vi "EXA_Get_Marker_Value.vi"(8 "error in":errorcluster, 10 "Marker\nNumber":i32, 11 "VISA resource name":refnum<visa-resource-name>) -> (0 "error out":errorcluster, 1 "Amplitude (dBm)":dbl, 2 "Frequency (Hz)":dbl, 3 "VISA resource name":refnum<visa-resource-name>)   [LabVIEW 2016]
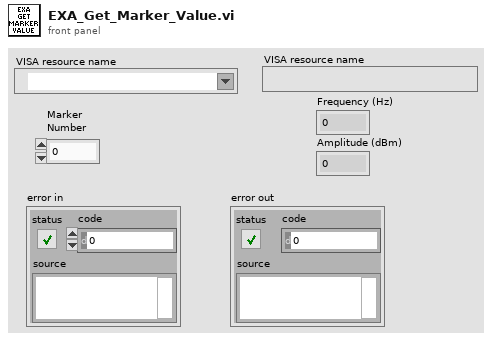
[diagram p1: front panel]
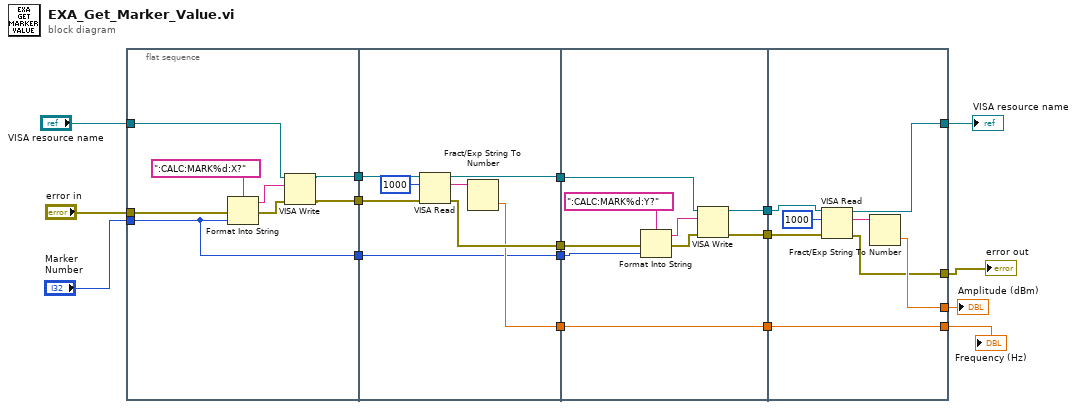
[diagram p0: block diagram]
diagram:
  n1 = flat-sequence {
    tunnel: "VISA resource name" -> [w25]
    tunnel: "Marker\nNumber" -> [w18]
    tunnel: "error in" -> [w21]
    tunnel: [w20] -> w14
    tunnel: [w19] -> w13
    tunnel: [w18] -> w8
    tunnel: w14 -> [w31]
    tunnel: w13 -> [w30]
    tunnel: [w29] -> w12
    tunnel: [w28] -> w11
    tunnel: [w27] -> w10
    tunnel: [w26] -> w9
    tunnel: w8 -> [w26]
    tunnel: w12 -> [w38]
    tunnel: w11 -> [w36]
    tunnel: w10 -> [w42]
    tunnel: w9 -> [w37]
    tunnel: [w42] -> w7
    tunnel: [w35] -> w6
    tunnel: [w34] -> w5
    tunnel: [w50] -> w1
    tunnel: w7 -> [w50]
    tunnel: w6 -> [w46]
    tunnel: w5 -> [w47]
    tunnel: [w45] -> w4
    tunnel: [w44] -> w2
    tunnel: [w43] -> w3
    frame #0 {
      n2 = Format Into String(format string=":CALC:MARK%d:X?", error in=w21, w18) -> (resulting string=w22:string, error out=w24:errorcluster)  [unwired: 1 in]
      n3 = VISA Write(VISA resource name=w25, write buffer=w22, error in (no error)=w24) -> (VISA resource name out=w19:refnum<visa-resource-name>, error out=w20:errorcluster)  [unwired: 1 out]
    }
    frame #1 {
      n4 = VISA Read(VISA resource name=w30, byte count=u32 1000, error in (no error)=w31) -> (VISA resource name out=w28:refnum<visa-resource-name>, read buffer=w33:string, error out=w29:errorcluster)  [unwired: 1 out]
      n5 = Fract/Exp String To Number(string=w33) -> (number=w27:dbl)  [unwired: 3 in, 1 out]
    }
    frame #2 {
      n6 = Format Into String(format string=":CALC:MARK%d:Y?", error in=w38, w37) -> (resulting string=w41:string, error out=w39:errorcluster)  [unwired: 1 in]
      n7 = VISA Write(VISA resource name=w36, write buffer=w41, error in (no error)=w39) -> (VISA resource name out=w34:refnum<visa-resource-name>, error out=w35:errorcluster)  [unwired: 1 out]
    }
    frame #3 {
      n8 = VISA Read(VISA resource name=w47, byte count=u32 1000, error in (no error)=w46) -> (VISA resource name out=w45:refnum<visa-resource-name>, read buffer=w48:string, error out=w43:errorcluster)  [unwired: 1 out]
      n9 = Fract/Exp String To Number(string=w48) -> (number=w44:dbl)  [unwired: 3 in, 1 out]
    }
  }
  "error out" <- w3
  "VISA resource name" <- w4
  "Amplitude (dBm)" <- w2
  "Frequency (Hz)" <- w1
